vi "Begin.vi"() -> (0 "error out":errorcluster)   [LabVIEW 2015]
doc: "Called before other user functions, this VI is expected to open initial I/O refnums, load in file data, and do all program initialization. Notice that the <B>error out</B> terminal is simply used for data flow. Wiring it to other structures or subVIs ensures that this VI runs first."
uses:
  <vilib>/Rock Robotics/WPI/DriverStation/WPI_DriverStationRobotMode2.ctl
  Device Refnums.ctl
  <vilib>/Rock Robotics/WPI/Joystick/WPI_JoystickDeviceEnum.ctl
  <vilib>/Rock Robotics/SystemInterfaces/DIO/FPGA_DIOPWMChannel.ctl
  <vilib>/Rock Robotics/WPI/SafetyOutput/WPI_SafetyOutputConfigMenu.ctl
  <vilib>/Rock Robotics/SystemInterfaces/DIO/FPGA_DIOChannel.ctl
  <vilib>/Rock Robotics/WPI/Encoder/WPI_EncoderType.ctl
  <vilib>/Rock Robotics/SystemInterfaces/AI/FPGA_AIChannel.ctl
  <vilib>/Rock Robotics/WPI/CAN/TalonSRX/WPI_CANTalonSRX_APIControlMode.ctl
  <vilib>/Rock Robotics/WPI/Solenoid/WPI_SolenoidChannel.ctl
  Robot Global Data.vi
  <vilib>/Rock Robotics/WPI/Solenoid/WPI_SolenoidOpenSingle.vi
  <vilib>/Rock Robotics/WPI/Solenoid/WPI_SolenoidOpenDouble.vi
  <vilib>/Rock Robotics/WPI/Utilities/WPI_GetSetVariantRefNum.vi
  <vilib>/Rock Robotics/WPI/MotorControl/WPI_MotorControlOpenCANTalonSRX.vi
  <vilib>/Rock Robotics/WPI/Counter/WPI_CounterDigitalInputToDigitalSource.vi
  <vilib>/Rock Robotics/WPI/Switch/WPI_SwitchOpenLimit.vi
  <vilib>/Rock Robotics/WPI/Ultrasonic/WPI_SonarMB1010DigitalOpen.vi
  <vilib>/Rock Robotics/WPI/Ultrasonic/WPI_SonarMB1010DigRefNum Registry Set.vi
  <vilib>/Rock Robotics/WPI/RobotDrive/WPI_RobotDriveOpen2MotorWithSPARK.vi
  <vilib>/Rock Robotics/WPI/MotorControl/WPI_MotorControlOpen VictorSP.vi
  ADIS16448-RoboRIO-Driver.git/trunk/LabVIEW/ADI MXP IMU/FRC ADI MXP IMU.lvlib
  <vilib>/Rock Robotics/WPI/MotorControl/WPI_MotorControlOpen Victor.vi
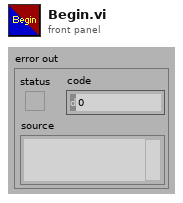
[diagram p1: front panel]
types:
  T1 = typedef "WPI_DriverStationRobotMode2.ctl" = enum16{"Autonomous Disabled", "Autonomous Enabled", "Teleop Disabled", "Teleop Enabled", "Disconnected", "Finish", "Test Disabled", "Test Enabled", "Emergency Stopped"}
  T2 = typedef "WPI_SolenoidChannel.ctl" = enum8{"Solenoid 0", "Solenoid 1", "Solenoid 2", "Solenoid 3", "Solenoid 4", "Solenoid 5", "Solenoid 6", "Solenoid 7", "Invalid"}
  T3 = typedef "Device Refnums.ctl" = string
  T4 = typedef "WPI_SolenoidDevRef.ctl" = cluster{"DevStatus":errorcluster, "Pneumatics Control Module":u8, "Forward Solenoid Channel":T2, "Reverse Solenoid Channel":T2}
  T5 = typedef "WPI_CompressorDevRef.ctl" = cluster{"DevStatus":errorcluster, "Pneumatics Control Module":u8}
  T6 = typedef "WPI_CANTalonSRX_APIControlMode.ctl" = enum8{"Percent VBus", "Speed", "Position", "Slave", "Unchanged / Invalid", "Voltage Compensation", "Current", "Motion Profile"}
  T7 = typedef "WPI_MotorControlDeviceRef.ctl" = cluster{"DeviceStatus":errorcluster, "Type":T8, "PWM":cluster{"PWM Channel":T9, "DeadBand":T10}, "CAN":cluster{"Device Number":u8, "Control Mode":T11, "Semaphore":T12, "Max Vout":dbl, "TalonSRX Control Mode":T6}, "Invert":bool}
  T8 = typedef "WPI_MotorControlType.ctl" = enum16{"PWM", "CAN", "CANTalonSRX"}
  T9 = typedef "FPGA_DIOPWMChannel.ctl" = enum8{"PWM 0", "PWM 1", "PWM 2", "PWM 3", "PWM 4", "PWM 5", "PWM 6", "PWM 7", "PWM 8", "PWM 9", "PWM MXP 0", "PWM MXP 1", "PWM MXP 2", "PWM MXP 3", "PWM MXP 4", "PWM MXP 5", "PWM MXP 6", "PWM MXP 7", "PWM MXP 8", "PWM MXP 9", "Invalid"}
  T10 = typedef "WPI_PWMDeadband.ctl" = cluster{"Name":string, "maxPositivePwm":i32, "minPositivePwm":i32, "centerPwm":i32, "maxNegativePwm":i32, "minNegativePwm":i32, "angularRange":u16}
  T11 = typedef "WPI_CANJaguar_ControlMode.ctl" = enum8{"Percent VBus", "Current", "Speed", "Position", "Voltage"}
  T12 = typedef "Semaphore RefNum" = refnum<k1>
  T13 = typedef "FPGA_AIChannel.ctl" = enum8{"AI 0", "AI 1", "AI 2", "AI 3", "AI MXP 0", "AI MXP 1", "AI MXP 2", "AI MXP 3", "Invalid"}
  T14 = typedef "WPI_AnalogChannelDevRef.ctl" = cluster{"DevStatus":errorcluster, "Analog Channel":T13}
  T15 = typedef "FRC ADI MXP IMU.lvlib/WPI_AnalogDevicesIMUInterruptDevRef.ctl" = cluster{"SimpleGyroDevRef":T16, "InterruptRef":T18}
  T16 = typedef "FRC ADI MXP IMU.lvlib/WPI_AnalogDevicesIMUDevRef.ctl" = cluster{"DevStatus":errorcluster, "Handle":i32, "SPI Bus":T17, "Device Found":bool, "Sample Rate":dbl, "Device Ready":bool, "Yaw Axis":enum16{"X", "Y", "Z"}, "AHRS Algorithm":enum16{"Complementary", "Madgwick"}}
  T17 = typedef "spi_bus.ctl" = enum16{"SPI On-Board, CS0", "SPI On-Board, CS1", "SPI On-Board, CS2", "SPI On-Board, CS3", "SPI MXP", "Invalid"}
  T18 = typedef "WPI_InterruptRef.ctl" = cluster{"DevStatus":errorcluster, "InterruptIndex":T19}
  T19 = typedef "FPGA_InterruptIndex.ctl" = enum8{"0", "1", "2", "3", "4", "5", "6", "7", "Invalid"}
  T20 = typedef "FPGA_DIOChannel.ctl" = enum8{"DIO 0", "DIO 1", "DIO 2", "DIO 3", "DIO 4", "DIO 5", "DIO 6", "DIO 7", "DIO 8", "DIO 9", "DIO MXP 0", "DIO MXP 1", "DIO MXP 2", "DIO MXP 3", "DIO MXP 4", "DIO MXP 5", "DIO MXP 6", "DIO MXP 7", "DIO MXP 8", "DIO MXP 9", "DIO MXP 10", "DIO MXP 11", "DIO MXP 12", "DIO MXP 13", "DIO MXP 14", "DIO MXP 15", "Invalid"}
  T21 = typedef "WPI_EncoderType.ctl" = enum16{"1x", "2x", "4x"}
  T22 = typedef "WPI_SonarMB1010DigitalDeviceRef.ctl" = cluster{"CounterDevRef":T23, "Scaling factor (s/in)":dbl}
  T23 = typedef "WPI_CounterDevRef.ctl" = cluster{"DevStatus":errorcluster, "CntIndex":T24}
  T24 = typedef "FPGA_CounterCtrSystemIndex.ctl" = enum8{"Ctr 0", "Ctr 1", "Ctr 2", "Ctr 3", "Ctr 4", "Ctr 5", "Ctr 6", "Ctr 7", "Invalid"}
  T25 = typedef "WPI_SwitchDevRef.ctl" = cluster{"DevStatus":errorcluster, "DIO Channel":T20, "CntIndex":T24, "Normally Closed":bool}
  T26 = typedef "WPI_DigitalInputDevRef.ctl" = cluster{"DevStatus":errorcluster, "DIO Channel":T20}
  T27 = typedef "FPGA_CounterEncoderSourceConvertionLVSourceType.ctl" = cluster{"DevStatus":errorcluster, "AnalogTriggerMode?":bool, "DigitalMode":cluster{"DIO Channel":T28}, "AnalogTriggerMode":cluster{"AnalogTriggerIndex":T29, "OutputType":T30}}
  T28 = typedef "FPGA_DIODigitalSourceChannel.ctl" = enum8{"DIO 0", "DIO 1", "DIO 2", "DIO 3", "DIO 4", "DIO 5", "DIO 6", "DIO 7", "DIO 8", "DIO 9", "DIO MXP 0", "DIO MXP 1", "DIO MXP 2", "DIO MXP 3", "DIO MXP 4", "DIO MXP 5", "DIO MXP 6", "DIO MXP 7", "DIO MXP 8", "DIO MXP 9", "DIO MXP 10", "DIO MXP 11", "DIO MXP 12", "DIO MXP 13", "DIO MXP 14", "DIO MXP 15", "Disabled"}
  T29 = typedef "FPGA_AnalogTriggerIndex.ctl" = enum8{"Trig 0", "Trig 1", "Trig 2", "Trig 3", "Trig 4", "Trig 5", "Trig 6", "Trig 7", "Invalid"}
  T30 = typedef "FPGA_AnalogTriggerOutType.ctl" = enum16{"InWindow", "TriggerState", "Rising", "Falling"}
  T31 = typedef "WPI_EncoderDevRef.ctl" = cluster{"DevStatus":errorcluster, "EncoderIndex":T32, "CounterIndex":T24, "DistancePerCount":dbl, "Decoding Type":T21}
  T32 = typedef "FPGA_EncoderIdx.ctl" = enum8{"Enc 0", "Enc 1", "Enc 2", "Enc 3", "Enc 4", "Enc 5", "Enc 6", "Enc 7", "Invalid"}
  T33 = typedef "WPI_SafetyOutputConfigMenu.ctl" = enum16{"Enable", "Disable"}
  T34 = typedef "WPI_RobotDriveDevRef.ctl" = cluster{"DevStatus":errorcluster, "Motors[]":T7[], "Square Inputs":bool, "Max Output":dbl}
  T35 = typedef "WPI_JoystickDeviceEnum.ctl" = enum16{"USB 0", "USB 1", "USB 2", "USB 3", "USB 4", "USB 5"}
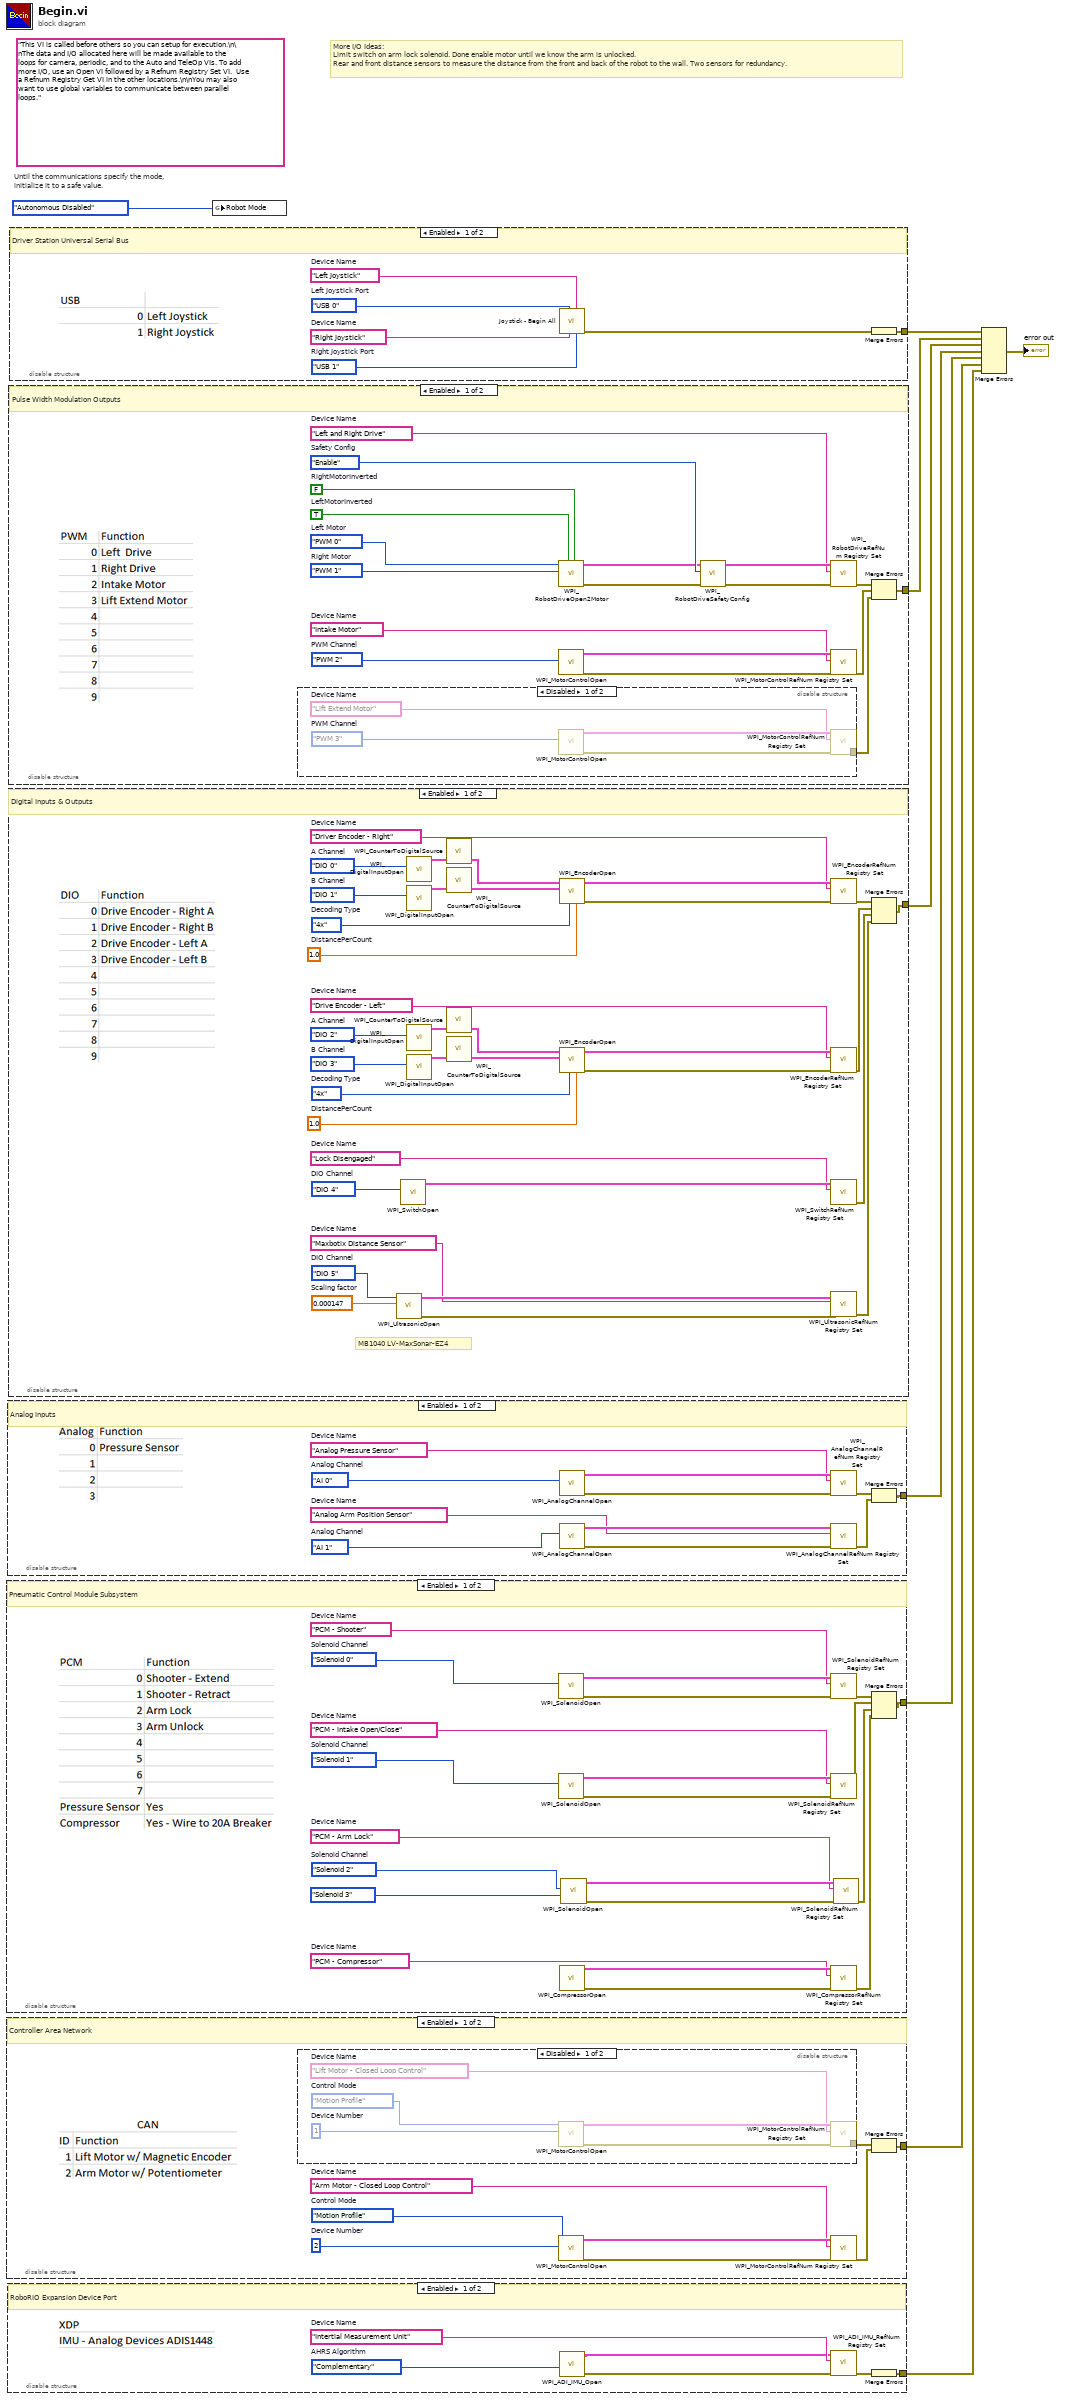
[diagram p0: block diagram]
diagram:
  (unwired) "This VI is called before others so you can setup for execution.\n\nThe data and I/O allocated here will be made available to the loops for camera, periodic, and to the Auto and TeleOp VIs. To add more I/O, use an Open VI followed by a Refnum Registry Set VI.  Use a Refnum Registry Get VI in the other locations.\n\nYou may also want to use global variables to communicate between parallel loops."
  # "More I/O Ideas:\nLimit switch on arm lock solenoid. Done enable motor until we know the arm is unlocked.\nRear and front distance sensors to measure the distance from the front and back of the robot to the wall. Two sensors for redundancy."
  # "Until the communications specify the mode,\ninitialize it to a safe value."
  n1 = disable-structure shown="Enabled" {
    disable-tunnel: [w22 _] -> w4
    frame Enabled {
      w11 = T3 "PCM - Intake Open/Close"  # Device Name
      w17 = WPI_SolenoidChannel."Solenoid 2"  # Solenoid Channel
      w18 = T3 "PCM - Compressor"  # Device Name
      w10 = T3 "PCM - Arm Lock"  # Device Name
      w19 = T3 "PCM - Shooter"  # Device Name
      w20 = WPI_SolenoidChannel."Solenoid 0"  # Solenoid Channel
      w21 = WPI_SolenoidChannel."Solenoid 1"  # Solenoid Channel
      # "Pneumatic Control Module Subsystem"
      n2 = call-poly <vilib>:"WPI_SolenoidOpen.vi"("Solenoid Channel"=w20) -> ("error out"=w27:errorcluster, "SolenoidDevRef"=w28:T4)  [unwired: 9 in]
      n3 = call-poly <vilib>:"WPI_SolenoidOpen.vi"("Solenoid Channel"=w21) -> ("error out"=w25:errorcluster, "SolenoidDevRef"=w26:T4)  [unwired: 9 in]
      n4 = call <vilib>:"WPI_CompressorOpen.vi"() -> ("CompressorDevRef"=w29:T5, "error out"=w30:errorcluster)  [unwired: 14 in]
      n5 = call-poly <vilib>:"WPI_SolenoidOpen.vi"("Reverse Solenoid Channel"=WPI_SolenoidChannel."Solenoid 3", "Forward Solenoid Channel"=w17) -> ("error out"=w16:errorcluster, "SolenoidDevRef"=w15:T4)  [unwired: 8 in]
      n6 = call <vilib>:"WPI_SolenoidRefNum Registry Set.vi"("error in (no error)"=w27, "refnum name"=w19, "SolenoidDevRef"=w28) -> ("error out"=w24:errorcluster)  [unwired: 7 in, 1 out]
      n7 = call <vilib>:"WPI_SolenoidRefNum Registry Set.vi"("error in (no error)"=w25, "refnum name"=w11, "SolenoidDevRef"=w26) -> ("error out"=w23:errorcluster)  [unwired: 7 in, 1 out]
      n8 = call <vilib>:"WPI_CompressorRefNum Registry Set.vi"("error in (no error)"=w30, "refnum name"=w18, "CompressorDevRef"=w29) -> ("error out"=w14:errorcluster)  [unwired: 7 in, 1 out]
      n9 = call <vilib>:"WPI_SolenoidRefNum Registry Set.vi"("error in (no error)"=w16, "refnum name"=w10, "SolenoidDevRef"=w15) -> ("error out"=w13:errorcluster)  [unwired: 7 in, 1 out]
      n10 = Merge Errors(w24, w23, w13, w14) -> (w22:errorcluster)
    }
    frame Disabled {
    }
  }
  n11 = disable-structure shown="Enabled" {
    disable-tunnel: [w31 _] -> w3
    frame Enabled {
      w34 = T3 "Arm Motor - Closed Loop Control"  # Device Name
      w35 = u8 2  # Device Number
      w36 = WPI_CANTalonSRX_APIControlMode."Motion Profile"  # Control Mode
      # "Controller Area Network"
      n12 = disable-structure shown="Disabled" {
        disable-tunnel: [w39 _] -> w33
        frame Disabled {
          w40 = T3 "Lift Motor - Closed Loop Control"  # Device Name
          w41 = u8 1  # Device Number
          w42 = WPI_CANTalonSRX_APIControlMode."Motion Profile"  # Control Mode
          n13 = call-poly <vilib>:"WPI_MotorControlOpen.vi"("Device Number"=w41, "Control Mode"=w42) -> ("error out"=w43:errorcluster, "MotorControlDeviceRef"=w44:T7)  [unwired: 8 in]
          n14 = call <vilib>:"WPI_MotorControlRefNum Registry Set.vi"("error in (no error)"=w43, "refnum name"=w40, "MotorControlDevRef"=w44) -> ("error out"=w39:errorcluster)  [unwired: 7 in, 1 out]
        }
        frame Enabled {
        }
      }
      n15 = call-poly <vilib>:"WPI_MotorControlOpen.vi"("Device Number"=w35, "Control Mode"=w36) -> ("error out"=w37:errorcluster, "MotorControlDeviceRef"=w38:T7)  [unwired: 8 in]
      n16 = call <vilib>:"WPI_MotorControlRefNum Registry Set.vi"("error in (no error)"=w37, "refnum name"=w34, "MotorControlDevRef"=w38) -> ("error out"=w32:errorcluster)  [unwired: 7 in, 1 out]
      n17 = Merge Errors(w33, w32) -> (w31:errorcluster)
    }
    frame Disabled {
    }
  }
  n18 = disable-structure shown="Enabled" {
    disable-tunnel: [w51 _] -> w5
    frame Enabled {
      w45 = T3 "Analog Arm Position Sensor"  # Device Name
      w50 = FPGA_AIChannel."AI 1"  # Analog Channel
      w52 = T3 "Analog Pressure Sensor"  # Device Name
      w55 = FPGA_AIChannel."AI 0"  # Analog Channel
      # "Analog Inputs"
      n19 = call <vilib>:"WPI_AnalogChannelOpen.vi"("Analog Channel"=w55) -> ("error out"=w53:errorcluster, "AIDeviceRef"=w54:T14)  [unwired: 9 in]
      n20 = call <vilib>:"WPI_AnalogChannelOpen.vi"("Analog Channel"=w50) -> ("error out"=w49:errorcluster, "AIDeviceRef"=w48:T14)  [unwired: 9 in]
      n21 = call <vilib>:"WPI_AnalogChannelRefNum Registry Set.vi"("error in (no error)"=w53, "refnum name"=w52, "AIDeviceRef"=w54) -> ("error out"=w47:errorcluster)  [unwired: 7 in, 1 out]
      n22 = call <vilib>:"WPI_AnalogChannelRefNum Registry Set.vi"("error in (no error)"=w49, "refnum name"=w45, "AIDeviceRef"=w48) -> ("error out"=w46:errorcluster)  [unwired: 7 in, 1 out]
      n23 = Merge Errors(w47, w46) -> (w51:errorcluster)
    }
    frame Disabled {
    }
  }
  n24 = disable-structure shown="Enabled" {
    disable-tunnel: [w59 _] -> w2
    frame Enabled {
      w61 = T3 "Intertial Measurement Unit"  # Device Name
      w58 = enum16{"Complementary", "Madgwick"}."Complementary"  # AHRS Algorithm
      # "RoboRIO Expansion Device Port"
      n25 = call "WPI_ADI_IMU_Open.vi"("AHRS Algorithm"=w58) -> ("error out"=w56:errorcluster, "ADI IMU Interrupt DevRef"=w57:T15)  [unwired: 9 in]
      n26 = call "WPI_ADI_IMU_RefNum Registry Set.vi"("error in (no error)"=w56, "refnum name"=w61, "ADI IMU Interrupt DevRef"=w57) -> ("error out"=w60:errorcluster)  [unwired: 7 in, 1 out]
      n27 = Merge Errors(w60) -> (w59:errorcluster)
    }
    frame Disabled {
    }
  }
  n28 = disable-structure shown="Enabled" {
    disable-tunnel: [w72 _] -> w6
    frame Enabled {
      w63 = FPGA_DIOChannel."DIO 5"  # DIO Channel
      w64 = 0.000147  # Scaling factor
      w65 = T3 "Maxbotix Distance Sensor"  # Device Name
      w68 = T3 "Lock Disengaged"  # Device Name
      w71 = FPGA_DIOChannel."DIO 4"  # DIO Channel
      w75 = T3 "Drive Encoder - Left"  # Device Name
      w76 = T3 "Driver Encoder - Right"  # Device Name
      w77 = 1.0  # DistancePerCount
      w78 = 1.0  # DistancePerCount
      w79 = WPI_EncoderType."4x"  # Decoding Type
      w80 = WPI_EncoderType."4x"  # Decoding Type
      w83 = FPGA_DIOChannel."DIO 3"  # B Channel
      w84 = FPGA_DIOChannel."DIO 2"  # A Channel
      w91 = FPGA_DIOChannel."DIO 1"  # B Channel
      w92 = FPGA_DIOChannel."DIO 0"  # A Channel
      # "MB1040 LV-MaxSonar-EZ4"
      # "Digital Inputs & Outputs"
      n29 = call-poly <vilib>:"WPI_UltrasonicOpen.vi"("Scaling factor (s/in)"=w64, "DIO Channel"=w63) -> ("error out"=w66:errorcluster, "SonarMB1010DigitalDevRef"=w67:T22)  [unwired: 8 in]
      n30 = call-poly <vilib>:"WPI_SwitchOpen.vi"("DIO Channel"=w71) -> ("SwitchDevRef"=w70:T25)  [unwired: 9 in, 1 out]
      n31 = call <vilib>:"WPI_DigitalInputOpen.vi"("DIO Channel"=w92) -> ("DigitalInputDevRef"=w95:T26)  [unwired: 1 in, 9 out]
      n32 = call <vilib>:"WPI_DigitalInputOpen.vi"("DIO Channel"=w91) -> ("DigitalInputDevRef"=w94:T26)  [unwired: 1 in, 9 out]
      n33 = call <vilib>:"WPI_DigitalInputOpen.vi"("DIO Channel"=w84) -> ("DigitalInputDevRef"=w87:T26)  [unwired: 1 in, 9 out]
      n34 = call <vilib>:"WPI_DigitalInputOpen.vi"("DIO Channel"=w83) -> ("DigitalInputDevRef"=w86:T26)  [unwired: 1 in, 9 out]
      n35 = call-poly <vilib>:"WPI_CounterToDigitalSource.vi"("DigitalInputDevRef"=w95) -> ("Digital Source"=w96:T27)  [unwired: 6 out]
      n36 = call-poly <vilib>:"WPI_CounterToDigitalSource.vi"("DigitalInputDevRef"=w94) -> ("Digital Source"=w93:T27)  [unwired: 6 out]
      n37 = call-poly <vilib>:"WPI_CounterToDigitalSource.vi"("DigitalInputDevRef"=w87) -> ("Digital Source"=w88:T27)  [unwired: 6 out]
      n38 = call-poly <vilib>:"WPI_CounterToDigitalSource.vi"("DigitalInputDevRef"=w86) -> ("Digital Source"=w85:T27)  [unwired: 6 out]
      n39 = call <vilib>:"WPI_EncoderOpen.vi"("DistancePerCount"=w78, "Decoding Type"=w79, "BSource"=w93, "ASource"=w96) -> ("error out"=w90:errorcluster, "EncoderDevRef"=w89:T31)  [unwired: 4 in, 2 out]
      n40 = call <vilib>:"WPI_EncoderOpen.vi"("DistancePerCount"=w77, "Decoding Type"=w80, "BSource"=w85, "ASource"=w88) -> ("error out"=w82:errorcluster, "EncoderDevRef"=w81:T31)  [unwired: 4 in, 2 out]
      n41 = call <vilib>:"WPI_EncoderRefNum Registry Set.vi"("error in (no error)"=w90, "refnum name"=w76, "EncoderDevRef"=w89) -> ("error out"=w74:errorcluster)  [unwired: 7 in, 1 out]
      n42 = call <vilib>:"WPI_EncoderRefNum Registry Set.vi"("error in (no error)"=w82, "refnum name"=w75, "EncoderDevRef"=w81) -> ("error out"=w73:errorcluster)  [unwired: 7 in, 1 out]
      n43 = call <vilib>:"WPI_SwitchRefNum Registry Set.vi"("refnum name"=w68, "SwitchDevRef"=w70) -> ("error out"=w69:errorcluster)  [unwired: 8 in, 1 out]
      n44 = call-poly <vilib>:"WPI_UltrasonicRefNum Registry Set.vi"("error in (no error)"=w66, "refnum name"=w65, "SonarMB1010DigitalDevRef"=w67) -> ("error out"=w62:errorcluster)  [unwired: 7 in, 1 out]
      n45 = Merge Errors(w74, w73, w69, w62) -> (w72:errorcluster)
    }
    frame Disabled {
    }
  }
  n46 = disable-structure shown="Enabled" {
    disable-tunnel: [w97 _] -> w7
    frame Enabled {
      w101 = T3 "Intake Motor"  # Device Name
      w102 = T3 "Left and Right Drive"  # Device Name
      w105 = FPGA_DIOPWMChannel."PWM 2"  # PWM Channel
      w110 = WPI_SafetyOutputConfigMenu."Enable"  # Safety Config
      w111 = FPGA_DIOPWMChannel."PWM 1"  # Right Motor
      w112 = FPGA_DIOPWMChannel."PWM 0"  # Left Motor
      w113 = TRUE  # LeftMotorInverted
      w114 = FALSE  # RightMotorInverted
      # "Pulse Width Modulation Outputs"
      n47 = disable-structure shown="Disabled" {
        disable-tunnel: [w115 _] -> w99
        frame Disabled {
          w116 = T3 "Lift Extend Motor"  # Device Name
          w118 = FPGA_DIOPWMChannel."PWM 3"  # PWM Channel
          n48 = call-poly <vilib>:"WPI_MotorControlOpen.vi"("PWM Channel"=w118) -> ("error out"=w117:errorcluster, "MotorControlDeviceRef"=w119:T7)  [unwired: 9 in]
          n49 = call <vilib>:"WPI_MotorControlRefNum Registry Set.vi"("error in (no error)"=w117, "refnum name"=w116, "MotorControlDevRef"=w119) -> ("error out"=w115:errorcluster)  [unwired: 7 in, 1 out]
        }
        frame Enabled {
        }
      }
      n50 = call-poly <vilib>:"WPI_RobotDriveOpen2Motor.vi"("Right Motor Inverted"=w114, "Left Motor Inverted"=w113, "Right Motor"=w111, "Left Motor"=w112) -> ("error out"=w107:errorcluster, "RobotDriveDevRef"=w106:T34)  [unwired: 1 in, 5 out]
      n51 = call-poly <vilib>:"WPI_MotorControlOpen.vi"("PWM Channel"=w105) -> ("error out"=w103:errorcluster, "MotorControlDeviceRef"=w104:T7)  [unwired: 9 in]
      n52 = call <vilib>:"WPI_RobotDriveSafetyConfig.vi"("error in (no error)"=w107, "mode"=w110, "RobotDriveDevRef"=w106) -> ("error out"=w109:errorcluster, "RobotDriveDevRef"=w108:T34)  [unwired: 7 in]
      n53 = call <vilib>:"WPI_RobotDriveRefNum Registry Set.vi"("error in (no error)"=w109, "refnum name"=w102, "RobotDriveDevRef"=w108) -> ("error out"=w100:errorcluster)  [unwired: 1 in, 7 out]
      n54 = call <vilib>:"WPI_MotorControlRefNum Registry Set.vi"("error in (no error)"=w103, "refnum name"=w101, "MotorControlDevRef"=w104) -> ("error out"=w98:errorcluster)  [unwired: 7 in, 1 out]
      n55 = Merge Errors(w100, w98, w99) -> (w97:errorcluster)
    }
    frame Disabled {
    }
  }
  n56 = disable-structure shown="Enabled" {
    disable-tunnel: [w120 _] -> w8
    frame Enabled {
      w122 = T3 "Right Joystick"  # Device Name
      w123 = T3 "Left Joystick"  # Device Name
      w124 = WPI_JoystickDeviceEnum."USB 1"  # Right Joystick Port
      w125 = WPI_JoystickDeviceEnum."USB 0"  # Left Joystick Port
      # "Driver Station Universal Serial Bus"
      n57 = call "Joystick - Begin All.vi"("Right Joystick Port"=w124, "Left Joystick Name"=w123, "Right Joystick Name"=w122, "Left Joystick Port"=w125) -> ("error out"=w121:errorcluster)  [unwired: 7 in]
      n58 = Merge Errors(w121) -> (w120:errorcluster)
    }
    frame Disabled {
    }
  }
  n59 = global write "Robot Global Data.vi" "Robot Mode"(WPI_DriverStationRobotMode2."Autonomous Disabled" ("Robot Mode")) -> ()
  n60 = Merge Errors(w8, w7, w6, w5, w4, w3, w2) -> (→"error out":errorcluster)
